vi "test - API String Arguments Support(Variant).vi"(8 "error in (no error)":errorcluster, 11 "TestCase in":refnum<class "testcase-Supported-Datatype.lvclass">) -> (0 "error out":errorcluster, 3 "TestCase out":refnum<class "testcase-Supported-Datatype.lvclass">)   [LabVIEW 2017, in "testcase-Supported-Datatype.lvclass"]
uses:
  testcase-Supported-Datatype.lvclass
  <vilib>/addons/_JKI Toolkits/VI Tester/TestCase.llb/TestCase.lvclass
  API-String-Arugments-Support/API String Arguments Support.lvlib
  C:/Program Files (x86)/National Instruments/LabVIEW 2017/vi.lib/addons/_JKI Toolkits/VI Tester/TestCase.llb/TestCase.lvclass
panel:
  out "data":dbl[][](array[numeric])
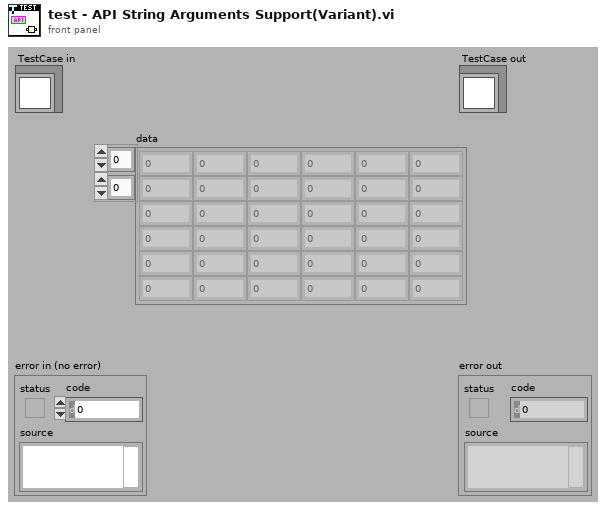
[diagram p1: front panel]
types:
  T1 = cluster{"Name":string, "Child":cluster{"Name":string}, "Bool":bool}[]
  T2 = cluster{"Name":string, "Child":cluster{"Name":string}, "Bool":bool}
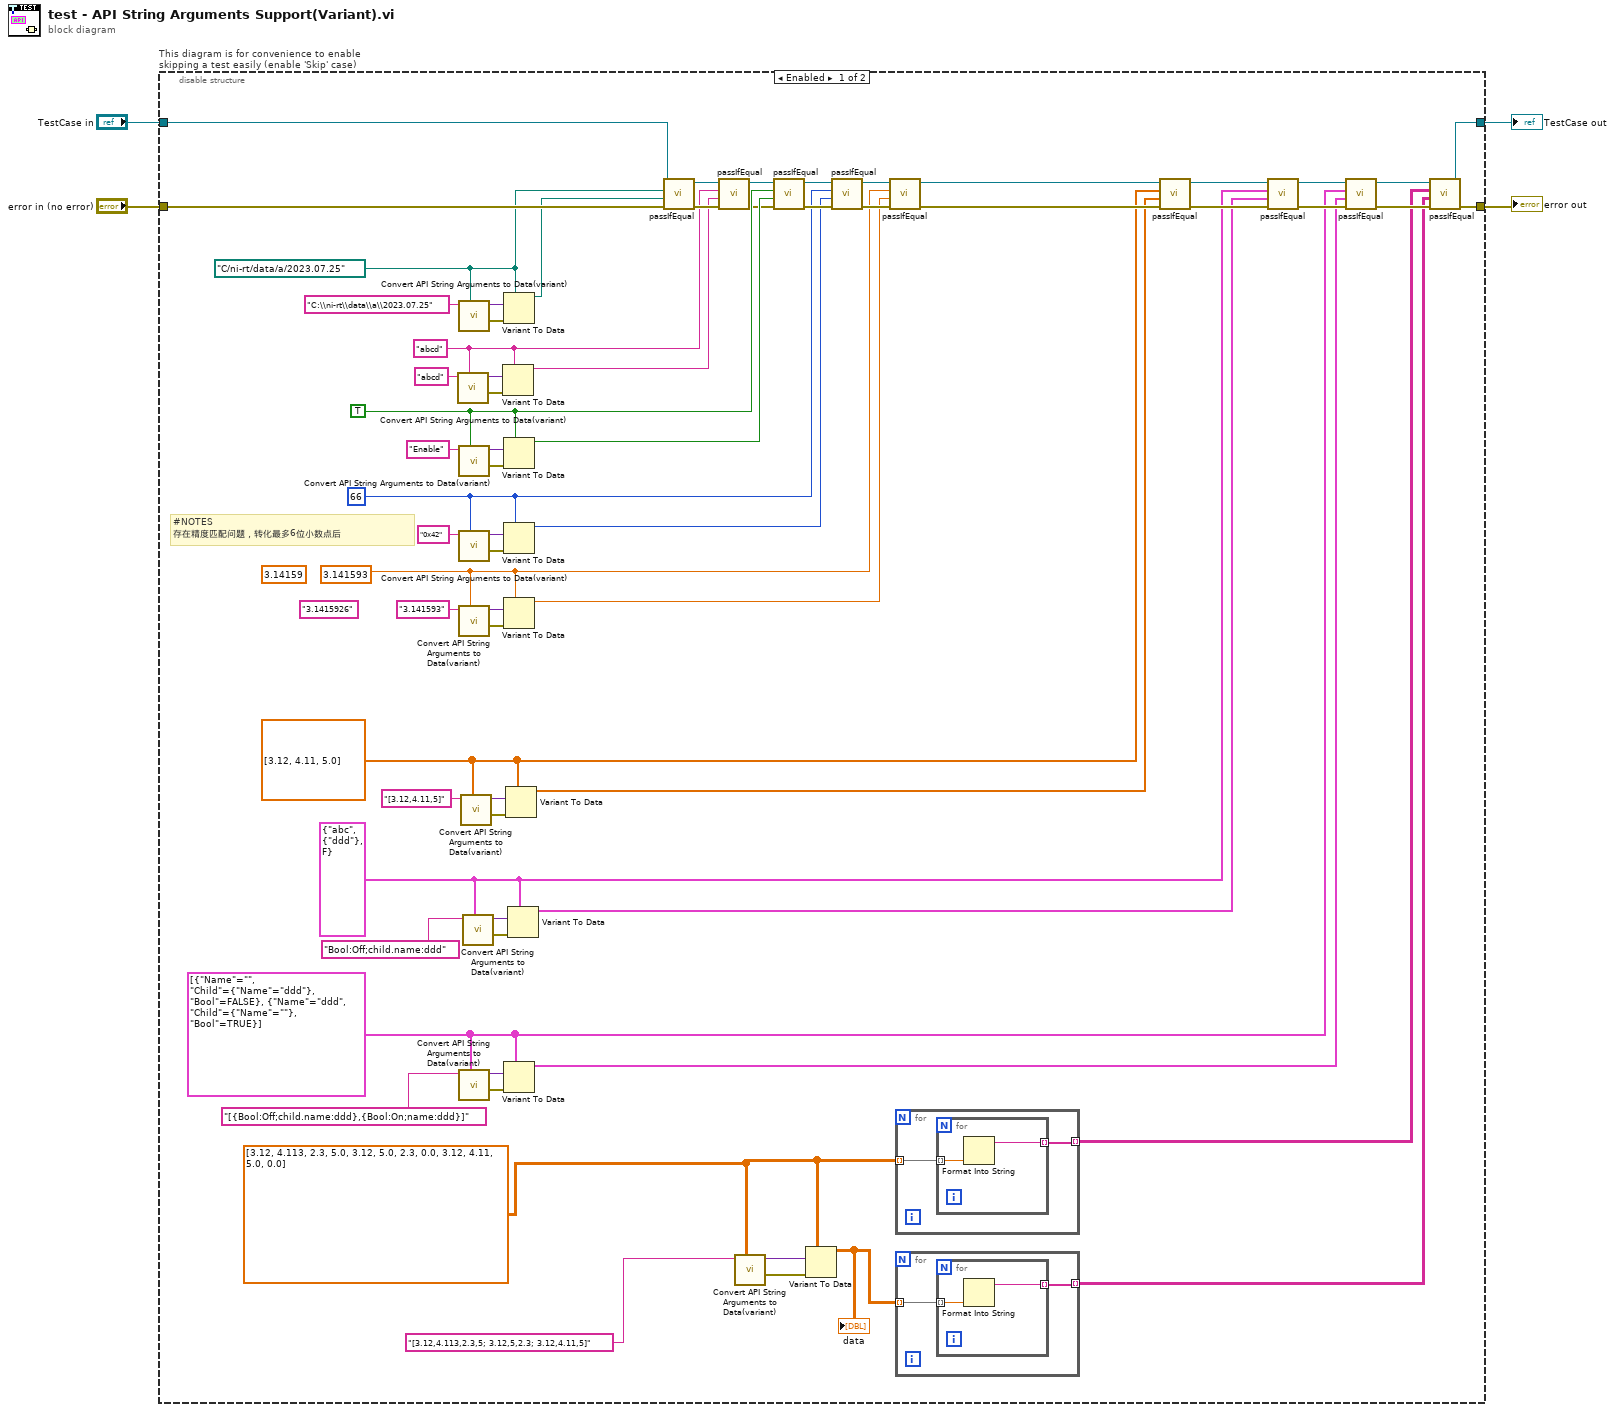
[diagram p0: block diagram]
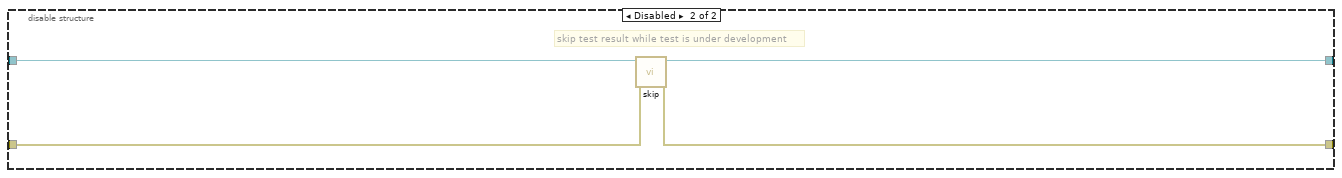
[diagram p2: hidden frame]
diagram:
  n1 = disable-structure "This diagram is for convenience to enable skipping a test easily (enable 'Skip' case)" shown="Enabled" {
    disable-tunnel: "TestCase in" -> [w71 w83]
    disable-tunnel: [w20 w81] -> w1
    disable-tunnel: [w21 w82] -> w3
    disable-tunnel: "error in (no error)" -> [w70 w80]
    frame Enabled {
      w5 = dbl[][] [[3.12, 4.113, 2.3, 5.0], [3.12, 5.0, 2.3, 0.0], [3.12, 4.11, 5.0, 0.0]] ("data")
      (unwired) "3.1415926" ("String")
      (unwired) 3.14159
      w10 = "abcd" ("String")
      w28 = T1 [{"Name"="", "Child"={"Name"="ddd"}, "Bool"=FALSE}, {"Name"="ddd", "Child"={"Name"=""}, "Bool"=TRUE}] ("Data 10")
      w35 = T2 {"Name"="abc", "Child"={"Name"="ddd"}, "Bool"=FALSE} ("Data 8")
      w42 = dbl[] [3.12, 4.11, 5.0] ("Data 4")
      w49 = 3.141593
      w56 = 66
      w63 = TRUE
      w19 = path "C:/ni-rt/data/a/2023.07.25" ("Data 9")
      # "#NOTES\n存在精度匹配问题，转化最多6位小数点后"
      n2 = call "Convert API String Arguments to Data(variant).vi"("Type"=w10, "String"="abcd") -> ("error"=w17:errorcluster, "Data"=w16:variant)  [unwired: 8 in]
      n3 = call "Convert API String Arguments to Data(variant).vi"("Type"=w19, "String"="C:\\ni-rt\\data\\a\\2023.07.25") -> ("error"=w69:errorcluster, "Data"=w68:variant)  [unwired: 8 in]
      n4 = call "Convert API String Arguments to Data(variant).vi"("Type"=w63, "String"="Enable") -> ("error"=w66:errorcluster, "Data"=w65:variant)  [unwired: 8 in]
      n5 = call "Convert API String Arguments to Data(variant).vi"("Type"=w56, "String"="0x42") -> ("error"=w59:errorcluster, "Data"=w60:variant)  [unwired: 8 in]
      n6 = call "Convert API String Arguments to Data(variant).vi"("Type"=w49, "String"="3.141593") -> ("error"=w54:errorcluster, "Data"=w53:variant)  [unwired: 8 in]
      n7 = call "Convert API String Arguments to Data(variant).vi"("Type"=w28, "String"="[{Bool:Off;child.name:ddd},{Bool:On;name:ddd}]") -> ("error"=w33:errorcluster, "Data"=w32:variant)  [unwired: 8 in]
      n8 = call "Convert API String Arguments to Data(variant).vi"("Type"=w42, "String"="[3.12,4.11,5]") -> ("error"=w45:errorcluster, "Data"=w44:variant)  [unwired: 8 in]
      n9 = call "Convert API String Arguments to Data(variant).vi"("Type"=w35, "String"="Bool:Off;child.name:ddd") -> ("error"=w38:errorcluster, "Data"=w39:variant)  [unwired: 8 in]
      n10 = Variant To Data(error in=w17, type=w10, Variant=w16) -> (data=w9:string)  [unwired: 1 out]
      n11 = Variant To Data(error in=w69, type=w19, Variant=w68) -> (data=w18:path)  [unwired: 1 out]
      n12 = Variant To Data(error in=w66, type=w63, Variant=w65) -> (data=w62:bool)  [unwired: 1 out]
      n13 = Variant To Data(error in=w59, type=w56, Variant=w60) -> (data=w55:i32)  [unwired: 1 out]
      n14 = Variant To Data(error in=w54, type=w49, Variant=w53) -> (data=w48:dbl)  [unwired: 1 out]
      n15 = Variant To Data(error in=w33, type=w28, Variant=w32) -> (data=w27:T1)  [unwired: 1 out]
      n16 = Variant To Data(error in=w45, type=w42, Variant=w44) -> (data=w41:dbl[])  [unwired: 1 out]
      n17 = Variant To Data(error in=w38, type=w35, Variant=w39) -> (data=w34:T2)  [unwired: 1 out]
      n18 = call-dynamic "passIfEqual.vi"("error in (no error)"=w70, "y"=w18, "x"=w19, "TestCase in"=w71) -> ("error out"=w13:errorcluster, "TestCase out"=w14:refnum<class "testcase-Supported-Datatype.lvclass">)  [unwired: 6 in]
      n19 = call-dynamic "passIfEqual.vi"("error in (no error)"=w13, "y"=w9, "x"=w10, "TestCase in"=w14) -> ("error out"=w11:errorcluster, "TestCase out"=w12:refnum<class "testcase-Supported-Datatype.lvclass">)  [unwired: 6 in]
      n20 = call "Convert API String Arguments to Data(variant).vi"("Type"=w5, "String"="[3.12,4.113,2.3,5; 3.12,5,2.3; 3.12,4.11,5]") -> ("error"=w24:errorcluster, "Data"=w25:variant)  [unwired: 8 in]
      n21 = call-dynamic "passIfEqual.vi"("error in (no error)"=w11, "y"=w62, "x"=w63, "TestCase in"=w12) -> ("error out"=w58:errorcluster, "TestCase out"=w57:refnum<class "testcase-Supported-Datatype.lvclass">)  [unwired: 6 in]
      n22 = Variant To Data(error in=w24, type=w5, Variant=w25) -> (data=w8:dbl[][])  [unwired: 1 out]
      "data" <- w8
      n23 = call-dynamic "passIfEqual.vi"("error in (no error)"=w58, "y"=w55, "x"=w56, "TestCase in"=w57) -> ("error out"=w50:errorcluster, "TestCase out"=w51:refnum<class "testcase-Supported-Datatype.lvclass">)  [unwired: 6 in]
      n24 = call-dynamic "passIfEqual.vi"("error in (no error)"=w50, "y"=w48, "x"=w49, "TestCase in"=w51) -> ("error out"=w47:errorcluster, "TestCase out"=w46:refnum<class "testcase-Supported-Datatype.lvclass">)  [unwired: 6 in]
      n25 = for {
        tunnel: w5 -> [w77] mode=indexing
        tunnel: [w76] -> w6 mode=indexing
        n26 = for {
          tunnel: w77 -> [w79] mode=indexing
          tunnel: [w78] -> w76 mode=indexing
          n27 = Format Into String(w79) -> (resulting string=w78:string)  [unwired: 3 in, 1 out]
        }
      }
      n28 = for {
        tunnel: w8 -> [w73] mode=indexing
        tunnel: [w72] -> w7 mode=indexing
        n29 = for {
          tunnel: w73 -> [w75] mode=indexing
          tunnel: [w74] -> w72 mode=indexing
          n30 = Format Into String(w75) -> (resulting string=w74:string)  [unwired: 3 in, 1 out]
        }
      }
      n31 = call-dynamic "passIfEqual.vi"("error in (no error)"=w47, "y"=w41, "x"=w42, "TestCase in"=w46) -> ("error out"=w36:errorcluster, "TestCase out"=w37:refnum<class "testcase-Supported-Datatype.lvclass">)  [unwired: 6 in]
      n32 = call-dynamic "passIfEqual.vi"("error in (no error)"=w36, "y"=w34, "x"=w35, "TestCase in"=w37) -> ("error out"=w29:errorcluster, "TestCase out"=w30:refnum<class "testcase-Supported-Datatype.lvclass">)  [unwired: 6 in]
      n33 = call-dynamic "passIfEqual.vi"("error in (no error)"=w29, "y"=w27, "x"=w28, "TestCase in"=w30) -> ("error out"=w22:errorcluster, "TestCase out"=w23:refnum<class "testcase-Supported-Datatype.lvclass">)  [unwired: 6 in]
      n34 = call-dynamic "passIfEqual.vi"("error in (no error)"=w22, "y"=w7, "x"=w6, "TestCase in"=w23) -> ("error out"=w21:errorcluster, "TestCase out"=w20:refnum<class "testcase-Supported-Datatype.lvclass">)  [unwired: 6 in]
    }
    frame Disabled {
      # "skip test result while test is under development"
      n35 = call <vilib>:"skip.vi"("error in (no error)"=w80, "TestCase in"=w83) -> ("error out"=w82:errorcluster, "TestCase out"=w81:refnum<class "testcase-Supported-Datatype.lvclass">)  [unwired: 8 in]
    }
  }
  "error out" <- w3
  "TestCase out" <- w1
